vi "Add Child Items to Tree.vi"(8 "error in (no error)":errorcluster, 10 "Polymorphic VI Type in":refnum<class "Polymorphic VI Type.lvclass">, 11 "Tree Ref in":refnum<vi>) -> (0 "error out":errorcluster, 2 "Polymorphic VI Type out":refnum<class "Polymorphic VI Type.lvclass">, 3 "Tree Ref out":refnum<vi>)   [LabVIEW 2020, in "Peek Window.lvlib" / "Polymorphic VI Type.lvclass"]
uses:
  Polymorphic VI Type.lvclass
  Polymorphic VI Type.lvclass/Polymorphic VI Type.ctl
  Standard VI Type/Standard VI Type.lvclass/Standard VI Type.ctl
  Symbols Enum.ctl
  Standard VI Type/Read Full Qualified Name.vi
  Implementation VI Type/Implementation VI Type.lvclass
  D:/Code/VI-Peek/source/Peek Window/VI Types/Standard VI Type/Standard VI Type.lvclass
  Peek Window.lvlib
  Standard VI Type/Standard VI Type.lvclass
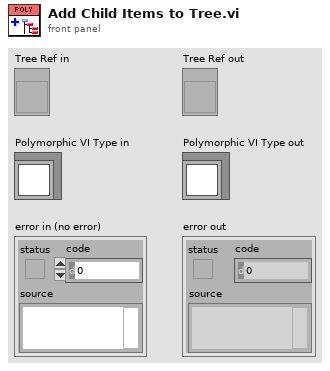
[diagram p1: front panel]
types:
  T1 = map{string, refnum<class "Implementation VI Type.lvclass">}
  T2 = cluster{"VIPath":path, "Menu Name":string, "Selector Name":string}[]
  T3 = typedef "Peek Window.lvlib/Symbols Enum.ctl" = enum16{"<Blank>", "Below Here Glyph", "VI", "Dynamic Dispatch VI", "Malleable VI", "Polymorphic VI", "Missing VI", "Express VI"}
  T4 = typedef "Peek Window.lvlib/Polymorphic VI Type.lvclass/Selected Item Enum.ctl" = enum16{"Polymorphic", "Instance"}
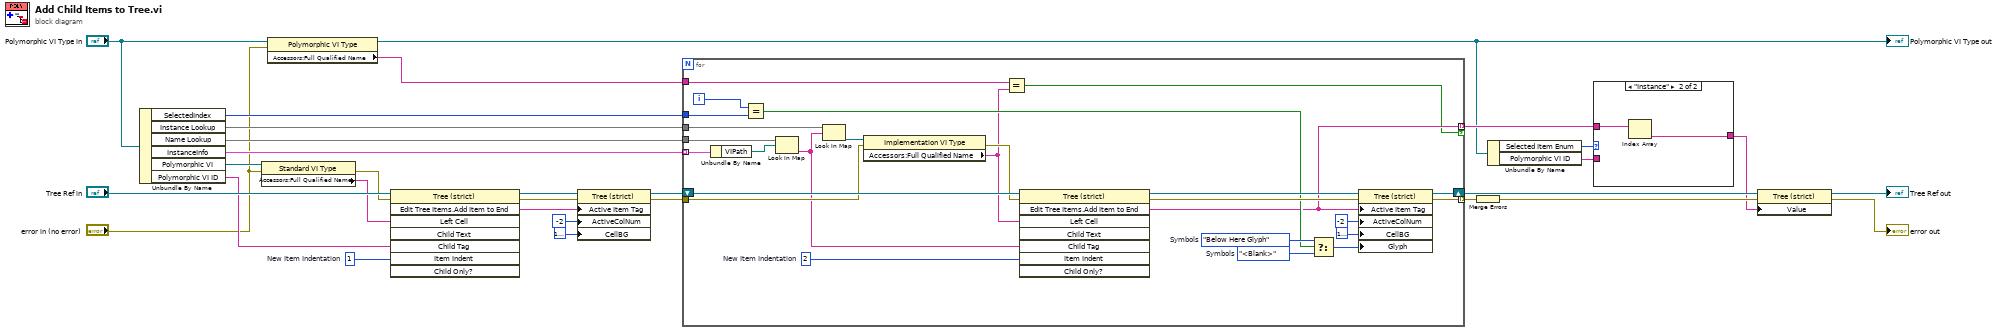
[diagram p0: block diagram]
diagram:
  w28 = 1  # New Item Indentation
  n1 = Unbundle By Name("Polymorphic VI Type in") -> ("SelectedIndex"=w13:i32, "Instance Lookup"=w12:T1, "Name Lookup"=w16:map{path, string}, "InstanceInfo"=w19:T2, "Polymorphic VI"=w30:refnum<class "Standard VI Type.lvclass">, "Polymorphic VI ID"=w15:string)
  n2 = property class="Standard VI Type"(reference=w30, error in="error in (no error)") -> (error out=w22:errorcluster, "Accessors:Full Qualified Name"=w14:string)  [unwired: 1 out]
  n3 = property class="Polymorphic VI Type"(reference="Polymorphic VI Type in", error in="error in (no error)") -> (reference out=w3:refnum<class "Polymorphic VI Type.lvclass">, "Accessors:Full Qualified Name"=w1:string)  [unwired: 1 out]
  "Polymorphic VI Type out" <- w3
  n4 = invoke class="Tree (strict)" method="Edit Tree Items.Add Item to End"(reference="Tree Ref in", error in=w22, "Left Cell"=w14, "Child Tag"=w15, "Item Indent"=w28) -> (reference out=w25:refnum<vi>, error out=w23:errorcluster, "Edit Tree Items:Add Item to End"=w24:string)  [unwired: 3 in, 5 out]
  n5 = property class="Tree (strict)"(reference=w25, error in=w23, "Active Item Tag"=w24, "ActiveColNum"=-2, "CellBG"=u32 16777238) -> (reference out=w20:refnum<vi>, error out=w21:errorcluster)
  n6 = for {
    tunnel: w21 -> [w37]
    shift-right: [w50] -> w10
    shift-left: w20 -> [w51]
    tunnel: w19 -> [w48] mode=indexing
    tunnel: [w49] -> w18 mode=indexing
    tunnel: w13 -> [w46]
    tunnel: w16 -> [w42]
    tunnel: w12 -> [w40]
    tunnel: [w34] -> w7 mode=indexing if=w31
    tunnel: w1 -> [w33]
    i -> [w47]
    w44 = Symbols_Enum."<Blank>"  # Symbols
    w45 = Symbols_Enum."Below Here Glyph"  # Symbols
    w52 = 2  # New Item Indentation
    n7 = Unbundle By Name(w48) -> ("VIPath"=w41:path)
    n8 = Equal?(x=w47, y=w46) -> (x = y?=w35:bool)
    n9 = Look In Map(map=w42, key=w41) -> (value=w36:string)  [unwired: 1 in, 1 out]
    n10 = Look In Map(map=w40, key=w36) -> (value=w39:refnum<class "Implementation VI Type.lvclass">)  [unwired: 1 in, 1 out]
    n11 = property class="Implementation VI Type"(reference=w39, error in=w37) -> (error out=w38:errorcluster, "Accessors:Full Qualified Name"=w32:string)  [unwired: 1 out]
    n12 = Equal?(x=w33, y=w32) -> (x = y?=w31:bool)
    n13 = invoke class="Tree (strict)" method="Edit Tree Items.Add Item to End"(reference=w51, error in=w38, "Left Cell"=w32, "Child Tag"=w36, "Item Indent"=w52) -> (reference out=w55:refnum<vi>, error out=w56:errorcluster, "Edit Tree Items:Add Item to End"=w34:string)  [unwired: 3 in, 5 out]
    n14 = Select(t=w45, s=w35, f=w44) -> (s? t:f=w43:T3)
    n15 = property class="Tree (strict)"(reference=w55, error in=w56, "Active Item Tag"=w34, "ActiveColNum"=-2, "CellBG"=u32 16777238, "Glyph"=w43) -> (reference out=w50:refnum<vi>, error out=w49:errorcluster)
  }
  n16 = Merge Errors(w18) -> (w17:errorcluster)
  n17 = Unbundle By Name(w3) -> ("Selected Item Enum"=w6:T4, "Polymorphic VI ID"=w4:string)
  n18 = case shown="\"Instance\"" w6 {
    tunnel: w7 -> [_ w59]
    tunnel: [w57 w58] -> w5
    tunnel: w4 -> [w57 _]
    frame "Polymorphic" {
    }
    frame "Instance" {
      n19 = Index Array(array=w59) -> (element=w58:string)  [unwired: 1 in]
    }
  }
  n20 = property class="Tree (strict)"(reference=w10, error in=w17, "Value"=w5) -> (reference out=→"Tree Ref out":refnum<vi>, error out=→"error out":errorcluster)
